vi "Omron Serial FINS-Check Sum.vi"(1 "Check String":string) -> (0 "FCS":string)   [LabVIEW 2016]
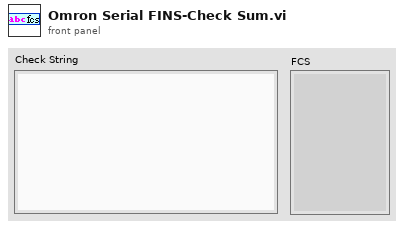
[diagram p1: front panel]
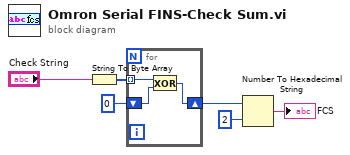
[diagram p0: block diagram]
diagram:
  n1 = String To Byte Array(string="Check String") -> (unsigned byte array=w4:u8[])
  n2 = for {
    tunnel: w4 -> [w9] mode=indexing
    shift-right: [w7] -> w2
    shift-left: u8 0 -> [w8]
    n3 = Exclusive Or(1:w8, 2:w9) -> (0:w7:u8)
  }
  n4 = Number To Hexadecimal String(1:i16 2 ("width (-)"), 2:w2) -> (0:→"FCS":string)
